vi "BuildResultsDirectoryPath.vi"(4 "Build Path(T)":bool, 6 "Test Type":string(combo), 7 "Lot#":string(combo), 8 "S/N":string, 9 "Chip Version":string(combo), 10 "Test":string(combo), 11 "Project":string(combo)) -> (1 "concatenated string":string, 3 "Sequence Result Directory":path)   [LabVIEW 2018]
uses:
  Initialize References/Sequence Globals.vi
panel:
  in  "Initial Path":path=path "C:/IdtATE/Results"
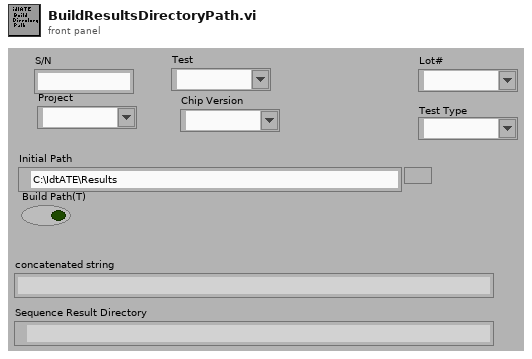
[diagram p1: front panel]
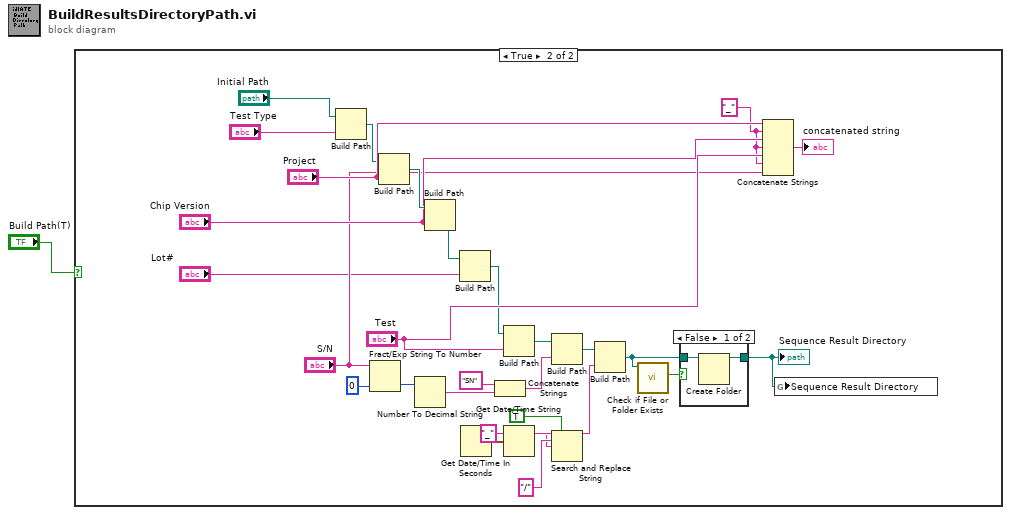
[diagram p0: block diagram]
diagram:
  n1 = case shown="True" "Build Path(T)" {
    frame False {
    }
    frame True {
      w9 = "_" ("string")
      n2 = Build Path(base path="Initial Path", name or relative path="Test Type") -> (appended path=w5:path)
      n3 = Fract/Exp String To Number(string="S/N", default (0 dbl)=i64 0 ("default (0 DBL)")) -> (number=w18:i64)  [unwired: 2 in, 1 out]
      n4 = Build Path(base path=w5, name or relative path="Project") -> (appended path=w20:path)
      n5 = Number To Decimal String(number=w18) -> (decimal integer string=w17:string)  [unwired: 1 in]
      n6 = Build Path(base path=w20, name or relative path="Chip Version") -> (appended path=w4:path)
      n7 = Build Path(base path=w4, name or relative path="Lot#") -> (appended path=w3:path)
      n8 = Get Date/Time In Seconds() -> (seconds since 1Jan1904=w24:timestamp)
      n9 = Concatenate Strings("SN" ("string"), w17) -> (w15:string)
      n10 = Build Path(base path=w3, name or relative path="Test") -> (appended path=w19:path)
      n11 = Get Date/Time String(seconds (now)=w24) -> (date string=w29:string)  [unwired: 2 in, 1 out]
      n12 = Build Path(base path=w19, name or relative path=w15) -> (appended path=w23:path)
      n13 = Search and Replace String(replace all?=TRUE ("replace all? (F)"), input string=w29, search string="/", replace string="_" ("replace string (\"\")")) -> (result string=w21:string)  [unwired: 4 in, 3 out]
      n14 = Build Path(base path=w23, name or relative path=w21) -> (appended path=w22:path)
      n15 = call <vilib>:"Check if File or Folder Exists.vi"("path"=w22) -> ("file or folder exists?"=w25:bool)  [unwired: 8 in, 2 out]
      n16 = case shown="False" w25 {
        tunnel: [w32 w33] -> w14
        tunnel: w22 -> [w31 w33]
        frame False {
          n17 = Create Folder(path (use dialog)=w31) -> (created path=w32:path)  [unwired: 2 in, 2 out]
        }
        frame True {
        }
      }
      "Sequence Result Directory" <- w14
      n18 = Concatenate Strings("Project", w9, "Chip Version", w9, "Test", w9, "S/N") -> (→"concatenated string":string)
      n19 = global write "Sequence Globals.vi" "Sequence Result Directory"(w14) -> ()
    }
  }
